vi "ReceiveTriggerCommand.vi"(8 "error in (no error)":errorcluster, 9 "Args":string[](array[string]), 10 "Command":string, 11 "TektronixDPOSimple in":refnum<class "TektronixDPO.lvclass">) -> (0 "error out":errorcluster, 2 "new commands":string, 3 "TektronixDPOSimple out":refnum<class "TektronixDPO.lvclass">)   [LabVIEW 2013, in "TektronixDPO.lvclass"]
uses:
  TektronixDPO.lvclass
  TektronixDPO.lvclass/TektronixDPO.ctl
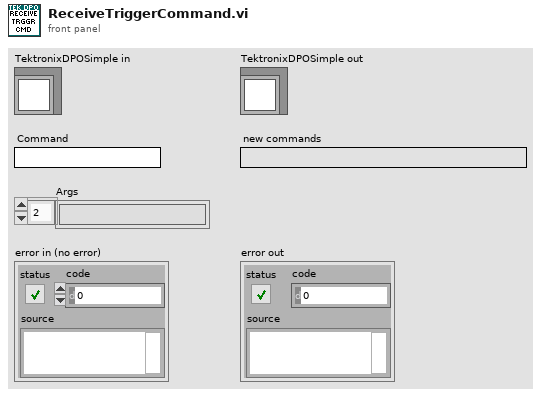
[diagram p1: front panel]
types:
  T1 = typedef "TriggerCluster.ctl" = cluster{"Mode":T2, "Source":T3, "Coupling":T4, "Slope":T5, "Low Level":dbl}
  T2 = typedef "Choice73.ctl" = enum16{"Immediate", "Analog Edge"}
  T3 = typedef "Choice74.ctl" = enum16{"Channel 1", "Channel 2", "Channel 3", "Channel 4", "AC Line", "Aux", "Digital Channel 0", "Digital Channel 1", "Digital Channel 2", "Digital Channel 3", "Digital Channel 4", "Digital Channel 5", "Digital Channel 6", "Digital Channel 7", "Digital Channel 8", "Digital Channel 9", "Digital Channel 10", "Digital Channel 11", "Digital Channel 12", "Digital Channel 13", "Digital Channel 14", "Digital Channel 15", "RF"}
  T4 = typedef "Choice75.ctl" = enum16{"DC", "HF Reject", "LF Reject", "Noise Reject", "AC"}
  T5 = typedef "Choice76.ctl" = enum16{"Rising", "Falling"}
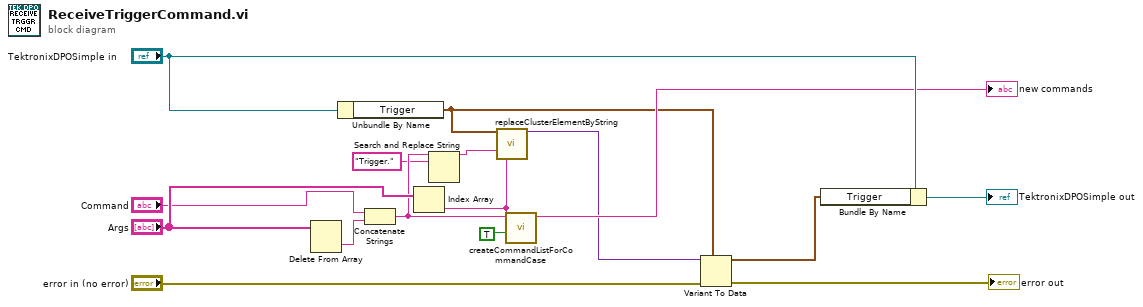
[diagram p0: block diagram]
diagram:
  n1 = Delete From Array(array="Args") -> (deleted portion=w8:string)  [unwired: 2 in, 1 out]
  n2 = Unbundle By Name("TektronixDPOSimple in") -> ("Trigger"=w6:T1)
  n3 = Concatenate Strings("Command", w8) -> (w3:string)
  n4 = Index Array(array="Args") -> (element=w5:string)  [unwired: 1 in]
  n5 = Search and Replace String(input string=w3, search string="Trigger.") -> (result string=w1:string)  [unwired: 6 in, 3 out]
  n6 = call "replaceClusterElementByString.vi"("cluster in"=w6, "Command"=w1, "setvalue"=w5) -> ("cluster out"=w7:variant)  [unwired: 10 in, 2 out]
  n7 = call "createCommandListForCommandCase.vi"("immediate Check (only once)"=TRUE, "setvalue"=w5, "command"=w3) -> ("new commands"=→"new commands":string)  [unwired: 8 in]
  n8 = Variant To Data(error in="error in (no error)", type=w6, Variant=w7) -> (data=w14:T1, error out=→"error out":errorcluster)
  n9 = Bundle By Name(cluster="TektronixDPOSimple in", "Trigger"=w14) -> (→"TektronixDPOSimple out":refnum<class "TektronixDPO.lvclass">)
